vi "BdcstWfrm.vi"(6 "Continuous":bool, 8 "error in (no error)":errorcluster, 9 "Waveforms":T1[](array[typedef]), 10 "Queue Array Reference In":refnum<queue>[](array[refnum]), 11 "ModuleAdmin":refnum<class "ModuleAdmin.lvclass">) -> (0 "error out":errorcluster, 1 "Continue":bool, 2 "Queue Array Reference Out":refnum<queue>[](array[refnum]))   [LabVIEW 2018, in "ScopePlugins.lvlib"]
uses:
  ScopePlugins.lvlib
  ScopeShared/Waveform.ctl
  <userlib>/NIST/ModuleAdminLib/ModuleAdmin/ModuleAdmin.lvclass
  Queue&Messages/clMessage.ctl
  ScopeShared/clEventType.ctl
  TypeDefs/QueueNames.ctl
  Queue&Messages/DequeueTypes.ctl
  ScopeShared/ScopeShared.lvlib
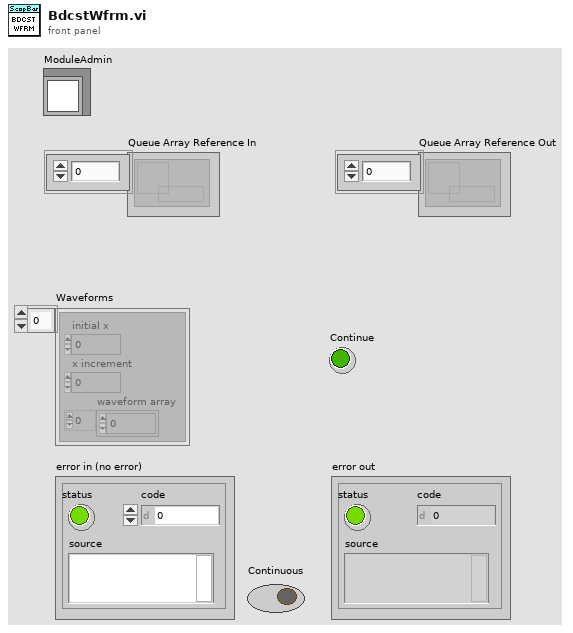
[diagram p1: front panel]
types:
  T1 = typedef "ScopeShared.lvlib/Waveform.ctl" = cluster{"initial x":dbl, "x increment":dbl, "waveform array":dbl[]}
  T2 = typedef "ScopePlugins.lvlib/DequeueTypes.ctl" = enum16{"PreviewQueue", "Dequeue"}
  T3 = typedef "ScopePlugins.lvlib/QueueNames.ctl" = enum16{"QMH", "Class ", "MA"}
  T4 = typedef "ScopeShared.lvlib/clEventType.ctl" = cluster{"ModuleID":i32, "Data":variant}
  T5 = typedef "ScopeShared.lvlib/clBroadcastEvents.ctl" = cluster{"DidInit":refnum<user-event>, "StatusUpdate":refnum<user-event>, "ErrorReport":refnum<user-event>, "DidStop":refnum<user-event>, "PathToINI":refnum<user-event>, "Handle":refnum<user-event>, "Model":refnum<user-event>, "Channels":refnum<user-event>, "Acquisition":refnum<user-event>, "Trigger":refnum<user-event>, "ExtAcquisition":refnum<user-event>, "Waveform":refnum<user-event>}
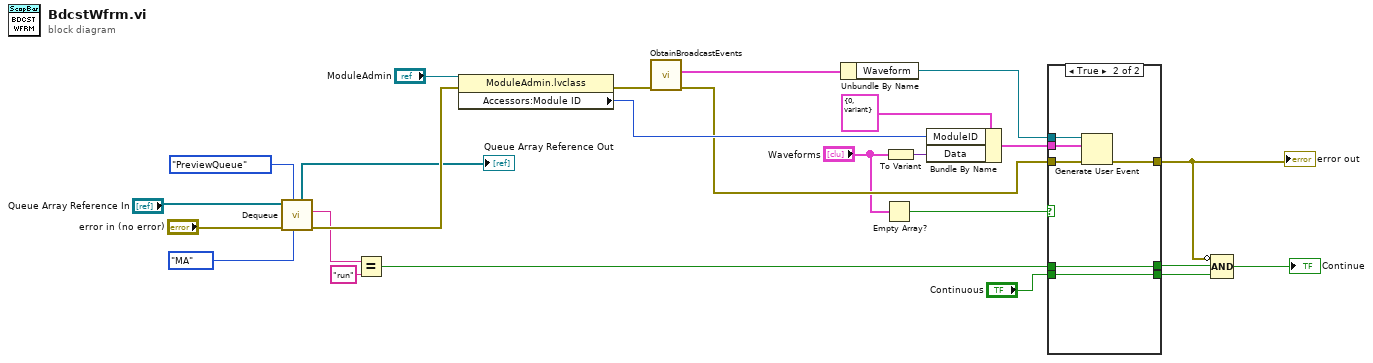
[diagram p0: block diagram]
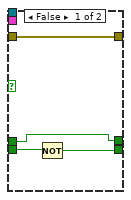
[diagram p2: hidden frame]
diagram:
  n1 = call "Dequeue.vi"("EnqueueType (QMH)"=QueueNames."MA", "DequeueType (PreviewQueue)"=DequeueTypes."PreviewQueue", "error in (no error)"="error in (no error)", "Queue Array Reference In"="Queue Array Reference In") -> ("error out"=w10:errorcluster, "Message"=w6:string, "Queue Array Reference Out"=→"Queue Array Reference Out":refnum<queue>[])  [unwired: 3 in, 2 out]
  n2 = Equal?(x=w6, y="run") -> (x = y?=w3:bool)
  n3 = property class="ModuleAdmin.lvclass"(reference="ModuleAdmin", error in=w10) -> (error out=w18:errorcluster, "Accessors:Module ID"=w19:i32)  [unwired: 1 out]
  n4 = call "ObtainBroadcastEvents.vi"("error in (no error)"=w18) -> ("error out"=w17:errorcluster, "clBroadcastEvents"=w25:T5)  [unwired: 9 in]
  n5 = Unbundle By Name(w25) -> ("Waveform"=w24:refnum<user-event>)
  n6 = Empty Array?(array="Waveforms") -> (empty?=w12:bool)
  n7 = To Variant(anything="Waveforms") -> (Variant=w22:variant)
  n8 = Bundle By Name(cluster=T4 {"ModuleID"=0, "Data"=variant} ("clEventType"), "ModuleID"=w19, "Data"=w22) -> (w21:T4)
  n9 = case shown="True" w12 {
    tunnel: w24 -> [_ w35]
    tunnel: w21 -> [_ w34]
    tunnel: [w29 w33] -> w9
    tunnel: w17 -> [w29 w32]
    tunnel: "Continuous" -> [w28 w31]
    tunnel: [w27 w31] -> w7
    tunnel: [w26 w30] -> w4
    tunnel: w3 -> [w26 w30]
    frame False {
      n10 = Not(x=w28) -> (.not. x?=w27:bool)
    }
    frame True {
      n11 = Generate User Event(user event=w35, event data cluster=w34, error in=w32) -> (error out=w33:errorcluster)  [unwired: 1 in, 1 out]
    }
  }
  "error out" <- w9
  n12 = Compound Arithmetic op=AND(invert w9, w4, w7) -> (→"Continue":bool)
